vi "S7_Close_TCP.vi"(8 "error in":errorcluster, 11 "TCP Connection Ref":refnum<k5>) -> (0 "error out":errorcluster)   [LabVIEW 2017, in "S7 TCP.lvlib"]
uses:
  S7 TCP.lvlib
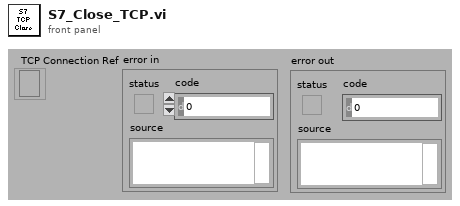
[diagram p1: front panel]
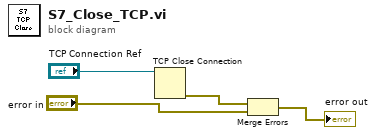
[diagram p0: block diagram]
diagram:
  n1 = TCP Close Connection(connection ID="TCP Connection Ref") -> (error out=w3:errorcluster)  [unwired: 1 in, 2 out]
  n2 = Merge Errors(w3, "error in") -> (→"error out":errorcluster)
